vi "NT Read Boolean.vi"(4 "options":T1={"Send All"=FALSE, "Keep Duplicates"=FALSE, "rate (hz)"=10}, 8 "error in":errorcluster, 9 "default value":bool, 11 "name":string="Boolean") -> (0 "error out":errorcluster, 1 "timestamp":u64, 3 "value":bool)   [LabVIEW 2025]
doc: "Read Boolean data from the subscribed topic. Returns an error and the default value if topic not present."
uses:
  <vilib>/Rock Robotics/Network Tables/NT SubscribeOptions.ctl
  <vilib>/Rock Robotics/Network Tables/NT Datatype.ctl
panel:
  in  "description":string="boolean"
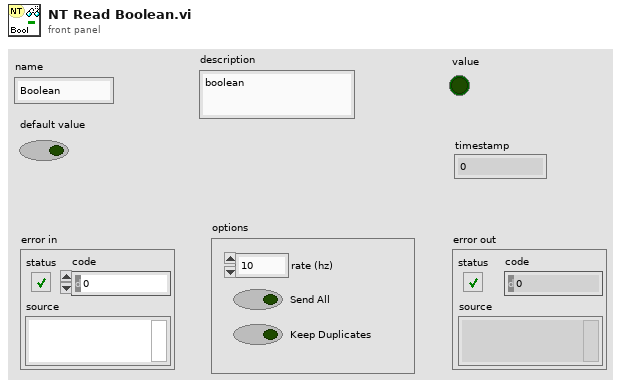
[diagram p1: front panel]
types:
  T1 = typedef "NT SubscribeOptions.ctl" = cluster{"Send All":bool, "Keep Duplicates":bool, "rate (hz)":u64}
  T2 = typedef "NT Datatype.ctl" = u32
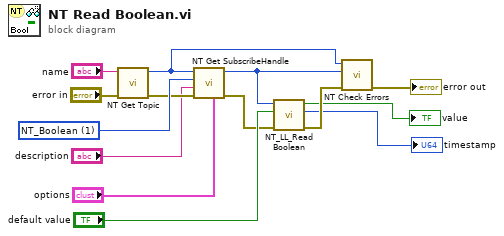
[diagram p0: block diagram]
diagram:
  w14 = T2 1 items=["NT_Unassigned"=0, "NT_Boolean"=1, "NT_Double"=2, "NT_String"=4, "NT_Raw"=8, "NT_BooleanArray"=16, "NT_DoubleArray"=32, "NT_StringArray"=64, "NT_RPC"=128, "NT_Integer"=256, "NT_Float"=512, "NT_IntegerArray"=1024, "NT_FloatArray"=2048] ("NT_Type")
  n1 = call <vilib>:"NT Get Topic.vi"("error in (no error)"="error in", "name"="name") -> ("error out"=w9:errorcluster, "topicHandle"=w3:u32)  [unwired: 8 in]
  n2 = call <vilib>:"NT Get SubscribeHandle.vi"("options"="options", "error in (no error)"=w9, "description"="description", "NT_Type"=w14, "topicHandle"=w3) -> ("error out"=w12:errorcluster, "subscribeHandle"=w4:u32)  [unwired: 5 in]
  n3 = call <vilib>:"NT_LL_Read Boolean.vi"("error in (no error)"=w12, "default value"="default value", "subscribeHandle"=w4) -> ("error out"=w6:errorcluster, "time"=→"timestamp":i64, "Boolean"=→"value":bool)  [unwired: 6 in]
  n4 = call <vilib>:"NT Check Errors.vi"("error in (no error)"=w6, "pubSubHandle"=w4, "topicHandle"=w3) -> ("error out"=→"error out":errorcluster)  [unwired: 8 in]
